vi "L0_RateScanBaseline_File_Appender.vi"(0 "file path (dialog if empty)":path, 1 "IPR":i64=63, 2 "Threshold":i32, 3 "CH":i8) -> ()   [LabVIEW 2012]
uses:
  <vilib>/Utility/file.llb/Write To Spreadsheet File (string).vi
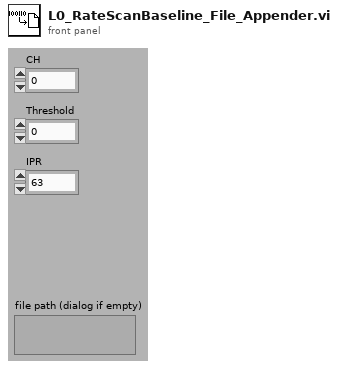
[diagram p1: front panel]
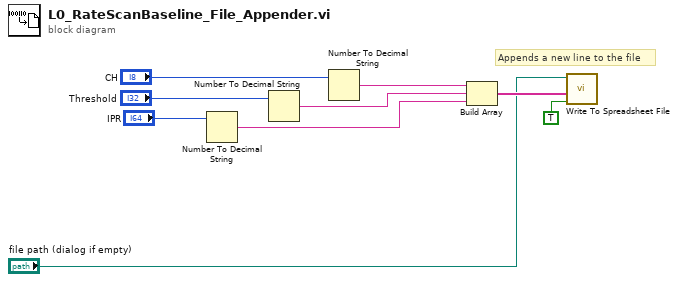
[diagram p0: block diagram]
diagram:
  # "Appends a new line to the file"
  n1 = Number To Decimal String(number="IPR") -> (decimal integer string=w7:string)  [unwired: 1 in]
  n2 = Number To Decimal String(number="Threshold") -> (decimal integer string=w8:string)  [unwired: 1 in]
  n3 = Number To Decimal String(number="CH") -> (decimal integer string=w9:string)  [unwired: 1 in]
  n4 = Build Array(w9, w8, w7) -> (w5:string[])
  n5 = call-poly <vilib>:"Write To Spreadsheet File.vi"("append to file? (new file:F)"=TRUE, "1D data"=w5, "file path (dialog if empty)"="file path (dialog if empty)") -> ()  [unwired: 5 in, 1 out]
